vi "04-nested_data_structures.vi"() -> ()   [LabVIEW 2018, in "LV-0mq-Julia_roundtrip-lib.lvlib"]
uses:
  LV-0mq-Julia_roundtrip-lib.lvlib
  Server or client state.ctl
  detailed error info.ctl
  StackFrame.ctl
  Commands.ctl
  c1a008e0-c205-4ae9-8ab0-5de19ea2baa8.vi
  c1a008e0-c205-4ae9-8ab0-5de19ea2baa8.vi/fb5c373d-d1bd-496d-9a76-88e6301317a3.vi
  c1a008e0-c205-4ae9-8ab0-5de19ea2baa8.vi/fb5c373d-d1bd-496d-9a76-88e6301317a3.vi/e57ee716-703a-4bb8-bc5c-1d233bfc9fd0.vi
  c1a008e0-c205-4ae9-8ab0-5de19ea2baa8.vi/fb5c373d-d1bd-496d-9a76-88e6301317a3.vi/d389da17-8964-463d-9351-1cd13380c13f.vi
  c1a008e0-c205-4ae9-8ab0-5de19ea2baa8.vi/fb5c373d-d1bd-496d-9a76-88e6301317a3.vi/54872663-7ef9-4399-95bb-da1de2cfd5e3.vi
  jl-scripts path.vi
  check ID validity.vi
  bindata_descr to JSON.vi
  check cluster field names.vi
  concat JSON.vi
  build request.vi
  Parse server response.vi
  log jl exceptions.vi
panel:
  out "returned value":T1
  in  "Argument":T2={"text_data"="hm?", "num_data"={"factor"=2, "num_arr"=[3.14, 2.72, 1.62]}} {"num_data"."num_arr" format="%#.2f"}
  in  "next":bool
  out "detailed error info":T3
  out "current error":errorcluster
  out "final error":errorcluster
  out "short err code":u8
  in  "stop":bool
  out "ZMQ timeout":bool
  out "Julia script file path":path
  out "temporary script path":path
  out "Jl Server state":T5
  # "Here the same (nested) data structure for the argument and returned value: for simplicity only."
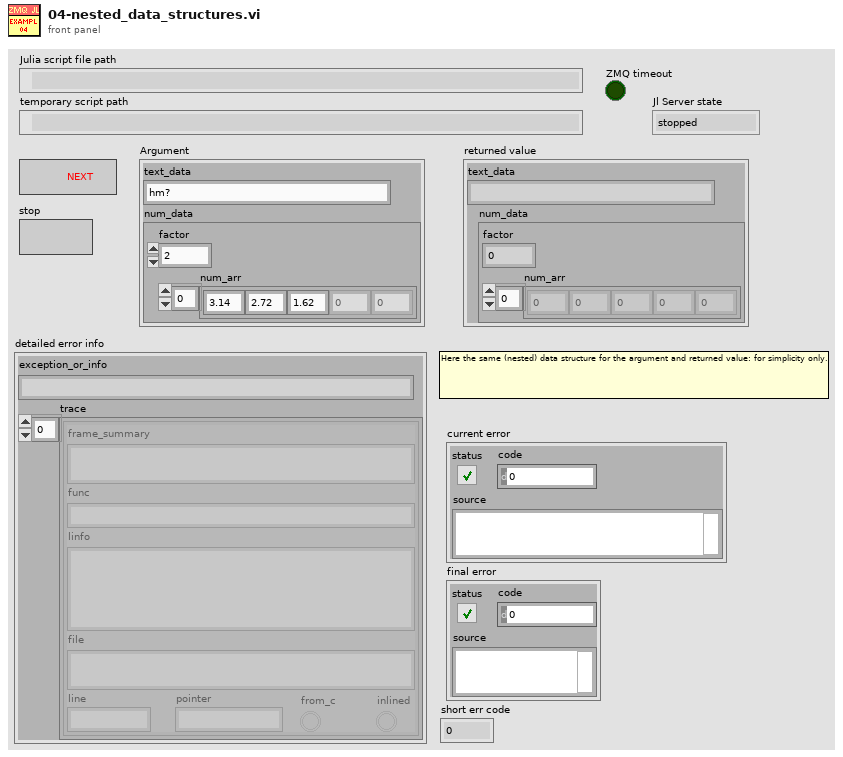
[diagram p1: front panel]
types:
  T1 = cluster{"text_data":string, "num_data":cluster{"factor":i32, "num_arr":dbl[]}}
  T2 = cluster{"text_data":string, "num_data":cluster{"factor":u32, "num_arr":dbl[]}}
  T3 = typedef "LV-0mq-Julia_roundtrip-lib.lvlib/detailed error info.ctl" = cluster{"exception_or_info":string, "trace":T4[]}
  T4 = typedef "LV-0mq-Julia_roundtrip-lib.lvlib/StackFrame.ctl" = cluster{"frame_summary":string, "func":string, "linfo":string, "file":string, "line":i32, "pointer":u64, "from_c":bool, "inlined":bool}
  T5 = typedef "LV-0mq-Julia_roundtrip-lib.lvlib/Server or client state.ctl" = enum16{"stopped", "running", "unknown"}
  T6 = typedef "LV-0mq-Julia_roundtrip-lib.lvlib/Commands.ctl" = enum16{"Start Jl-server & Init LV-client", "Send request & Get response ", "Stop Jl-server & Cleanup LV-client", "Cleanup LV-client", "Start Jl-server", "Stop Jl-server", "Init LV-Client", "Cleanup LV-Client", "(not allowed)", "Set LV Client state", "Set Jl Server state", "set ZMQ timeout", "read ZMQ timeout", "read-out state"}
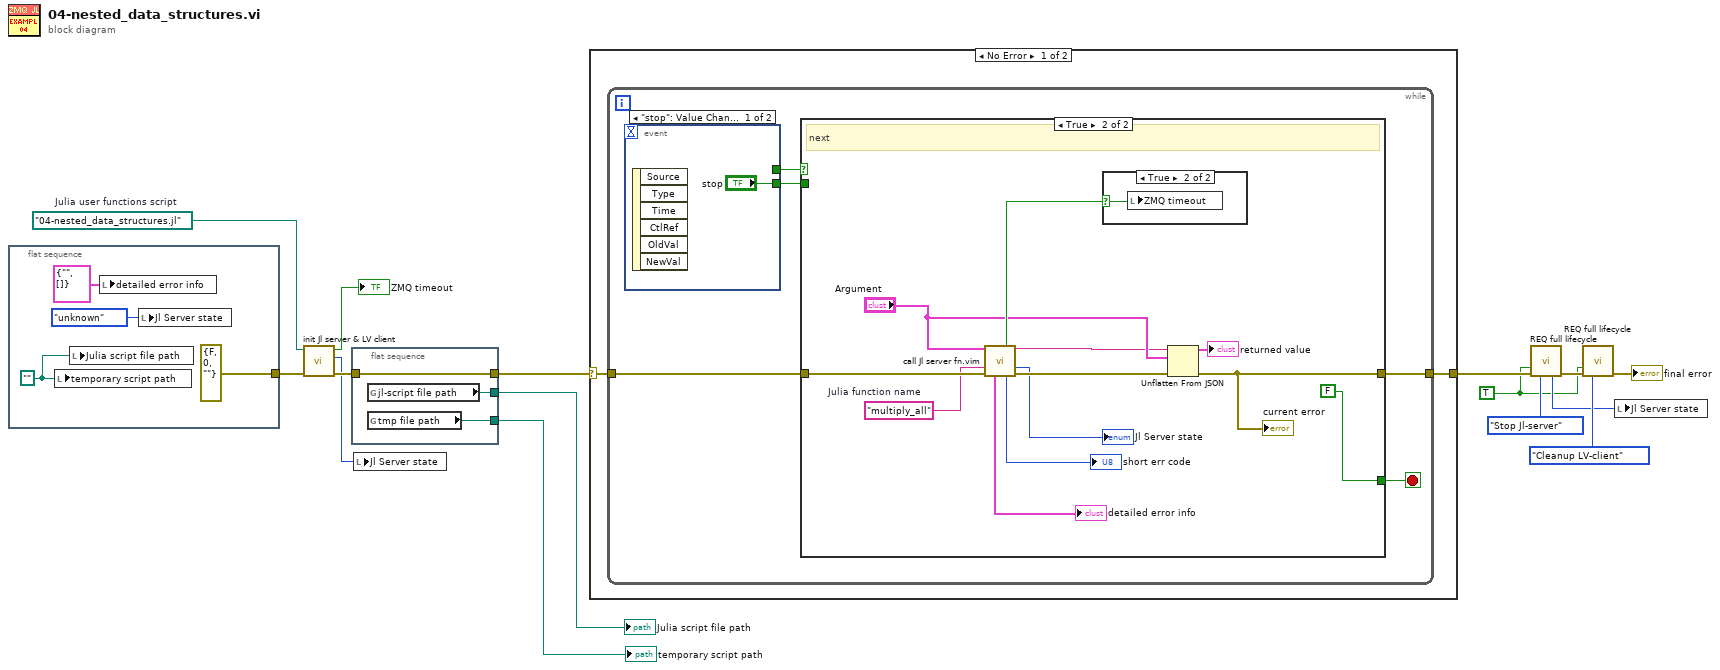
[diagram p0: block diagram]
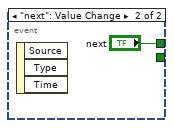
[diagram p2: hidden frame]
diagram:
  w1 = path "04-nested_data_structures.jl"  # Julia user functions script
  w6 = TRUE ("Force command")
  n1 = flat-sequence {
    tunnel: [errorcluster {"status"=FALSE, "code"=0, "source"=""} ("error in (no error)")] -> w5
    frame #0 {
      w16 = path ""
      n2 = local write "temporary script path"(w16) -> ()
      n3 = local write "Julia script file path"(w16) -> ()
      n4 = local write "detailed error info"(T3 {"exception_or_info"="", "trace"=[]} ("detailed error info")) -> ()
      n5 = local write "Jl Server state"(Server_or_client_state."unknown" ("Jl Server state out")) -> ()
    }
  }
  n6 = call "init Jl server & LV client.vi"("error in (no error)"=w5, "Julia user functions script"=w1) -> ("error out"=w4:errorcluster, "Jl Server state out"=w2:T5, "timeout?"=→"ZMQ timeout":bool)  [unwired: 7 in]
  n7 = flat-sequence {
    tunnel: [w22] -> w10
    tunnel: w4 -> [w22]
    tunnel: [w21] -> w8
    tunnel: [w20] -> w9
    frame #0 {
      n8 = global read "jl-scripts path.vi" "jl-script file path"() -> (w21:path)
      n9 = global read "jl-scripts path.vi" "tmp file path"() -> (w20:path)
    }
  }
  n10 = local write "Jl Server state"(w2) -> ()
  n11 = case shown="No Error" w10 {
    selector: w10 -> [w23 w47]
    tunnel: [w24 w47] -> w15
    frame No Error {
      n12 = while {
        tunnel: w23 -> [w28]
        tunnel: [w29] -> w24
        stop <- w26 stop-if-true
        n13 = event shown="[0] \"stop\": Value Change" {
          selector: _ -> [_ _]
          dyn-events: _ -> [_ _]
          timeout: _ -> [_ _]
          tunnel: [_ "next"] -> w27
          tunnel: ["stop" _] -> w25
          event "stop": Value Change {
            n14 = event-data() -> ()  [unwired: 1 in, 6 out]
          }
          event "next": Value Change {
            n15 = event-data() -> ()  [unwired: 1 in, 3 out]
          }
        }
        n16 = case shown="True" w27 {
          tunnel: [w33 w44] -> w29
          tunnel: w28 -> [w33 w42]
          tunnel: [w32 FALSE ("stop this VI only")] -> w26
          tunnel: w25 -> [w32 _]
          frame False {
            # "stop"
          }
          frame True {
            w35 = "multiply_all"  # Julia function name
            # "next"
            n17 = call "call Jl server fn.vim"("Arguments 1"="Argument", "fun2call"=w35, "error in (no error)"=w42) -> ("timeout?"=w37:bool, "JSON received"=w34:string, "Jl Server state out"=→"Jl Server state":T5, "detailed error info"=→"detailed error info":T3, "return code"=→"short err code":u8, "error out"=w41:errorcluster)  [unwired: 6 in, 1 out]
            n18 = case shown="True" w37 {
              selector: w37 -> [_ w46]
              frame False {
              }
              frame True {
                n19 = local write "ZMQ timeout"(w46) -> ()
              }
            }
            n20 = Unflatten From JSON(JSON string=w34, type and defaults="Argument", error in (no error)=w41) -> (value=→"returned value":T2, error out=w44:errorcluster)  [unwired: 4 in]
            "current error" <- w44
          }
        }
      }
    }
    frame Error {
    }
  }
  n21 = call "REQ full lifecycle.vi"("Force command"=w6, "error in"=w15, "command"=Commands."Stop Jl-server") -> ("Jl Server state out"=w7:T5, "error out"=w13:errorcluster)  [unwired: 6 in, 5 out]
  n22 = call "REQ full lifecycle.vi"("Force command"=w6, "error in"=w13, "command"=Commands."Cleanup LV-client") -> ("error out"=→"final error":errorcluster)  [unwired: 6 in, 6 out]
  n23 = local write "Jl Server state"(w7) -> ()
  "temporary script path" <- w9
  "Julia script file path" <- w8
